vi "fGetTransactions.vi"(11 "file path  2":path) -> (0 "Array":string[](array[string]))   [LabVIEW 2023]
uses:
  <vilib>/Utility/error.llb/Trim Whitespace One-Sided.vi
panel:
  out "size(s) All":i32
  out "size(s)":i32
  out "element":string
  out "Array 3":string[](array[string])
  in  "Transaction Type":T1(ring)
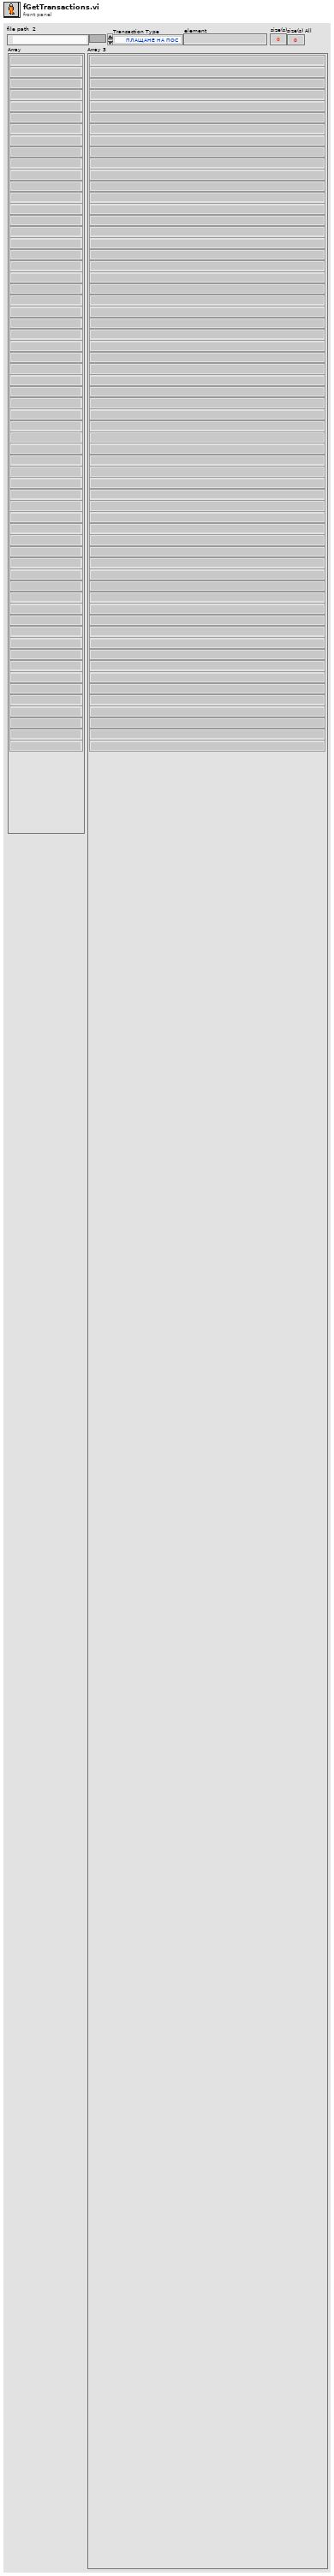
[diagram p1: front panel]
types:
  T1 = enum16{"ПЛАЩАНЕ НА ПОС", "СБКО", "ТЕГЛЕНЕ", "ЗАЕМ", "BREZOVO", "VIVACOM", "ЕЛЕКТРОХОЛД", "ЕВН", "ЗАПЛАТА", "АВАНС", "НЕТ", "ТРАНСФЕР"}
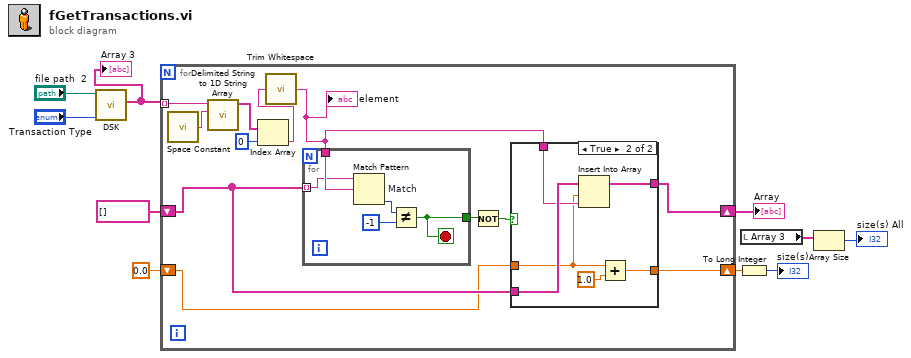
[diagram p0: block diagram]
diagram:
  n1 = call "DSK.vi"("Transaction Type"="Transaction Type", "file path"="file path  2") -> ("Array 3"=w10:string[])  [unwired: 6 in, 3 out]
  "Array 3" <- w10
  n2 = for {
    tunnel: w10 -> [w22] mode=indexing
    shift-right: [w13] -> w5
    shift-left: string[] [] -> [w16]
    shift-right: [w15] -> w1
    shift-left: 0.0 ("y") -> [w14]
    n3 = call <vilib>:"Space Constant.vi"() -> ("String"=w21:string)
    n4 = call <vilib>:"Delimited String to 1D String Array.vi"("delimiter"=w21, "delimited string"=w22) -> ("string array"=w20:string[])  [unwired: 9 in]
    n5 = Index Array(array=w20, index=0) -> (element=w12:string)
    n6 = call <vilib>:"Trim Whitespace.vi"("string"=w12) -> ("trimmed string"=w11:string)  [unwired: 1 in]
    "element" <- w11
    n7 = for {
      tunnel: w11 -> [w35]
      tunnel: w16 -> [w34] mode=indexing
      tunnel: [w31] -> w18
      stop <- w31 stop-if-true
      n8 = Match Pattern "Match"(string=w34, regular expression=w35) -> (offset past match=w33:i32)  [unwired: 1 in, 3 out]
      n9 = Not Equal?(x=w33, y=-1) -> (x != y?=w31:bool)
    }
    n10 = Not(x=w18) -> (.not. x?=w17:bool)
    n11 = case shown="True" w17 {
      tunnel: w16 -> [w23 w30]
      tunnel: w11 -> [_ w29]
      tunnel: [w24 w28] -> w15
      tunnel: w14 -> [w24 w26]
      tunnel: [w23 w25] -> w13
      frame False {
      }
      frame True {
        n12 = Insert Into Array(array=w30, index=w26, new element=w29) -> (w25:string[])
        n13 = Add(x=w26, y=1.0) -> (x+y=w28:dbl)
      }
    }
  }
  "Array" <- w5
  n14 = To Long Integer(number=w1) -> (32bit integer=→"size(s)":i32)
  n15 = local read "Array 3"() -> (w3:string[])
  n16 = Array Size(array=w3) -> (size(s)=→"size(s) All":i32)
